vi "Autonomous.vi"() -> ()   [LabVIEW 2025]
doc: "This VI starts when autonomous period begins, and will automatically be terminated when it ends. You can carry out timed or sensor driven operations directly to I/O or to subsystems without needing to return to the caller."
uses:
  <vilib>/Rock Robotics/WPI/ThirdParty/Phoenix-LabVIEW/Pigeon IMU/CTRE_PigeonIMU_TareType.ctl
  <vilib>/Rock Robotics/WPI/Utilities/WPI_GetSetVariantRefNum.vi
  <vilib>/Rock Robotics/Network Tables/NT Read String.vi
  Framework/Robot Global Data.vi
  <vilib>/Rock Robotics/Network Tables/NT Read String Array.vi
  <vilib>/Utility/file.llb/Read Delimited Spreadsheet (string).vi
  <vilib>/Rock Robotics/Network Tables/NT Write Numeric Array.vi
panel:
  in  "Is Blue Alliance?":bool
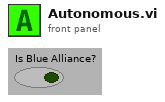
[diagram p1: front panel]
types:
  T1 = typedef "WPI_JoystickDevRef.ctl" = cluster{"Device":T2}
  T2 = typedef "WPI_JoystickDeviceEnum.ctl" = enum16{"USB 0", "USB 1", "USB 2", "USB 3", "USB 4", "USB 5"}
  T3 = cluster{"Field Centric":bool, "Auto Corretion":bool, "Theta Align":bool}
  T4 = typedef "CTRE_PigeonIMU_TareType.ctl" = u8
  T5 = typedef "Robot Velocities.ctl" = cluster{"X Velocity":dbl, "Y Velocity":dbl, "Rotational \nVelocity":dbl}
  T6 = typedef "Single Cmd Info.ctl" = cluster{"Name":string, "CPTM.DataType":variant, "All Control Values Variant":cluster{"Name":string, "Variant Data":variant}[], "icon full":T7, "icon scaled":T7, "Path":path, "Subsystem Color":u32}
  T7 = typedef "imagedata.ctl" = cluster{"image type":i32, "image depth":i32, "image":u8[], "mask":u8[], "colors":u32[], "Rectangle":cluster{"left":i16, "top":i16, "right":i16, "bottom":i16}}
  T8 = cluster{"Name":string, "vi reference":refnum<vi>, i32[], variant[]}
  T9 = cluster{dbl, "Command out":cluster{"Name":string, "vi reference":refnum<vi>, i32[], variant[]}}
  T10 = cluster{dbl, "Command out":cluster{"Name":string, "vi reference":refnum<vi>, i32[], variant[]}}[]
  T11 = cluster{"Velocities":T5[], "Positions":cluster{"x":dbl, "y":dbl, "th":dbl}[], cluster{dbl, "Command out":cluster{"Name":string, "vi reference":refnum<vi>, i32[], variant[]}}[], "Zero Velocity?":bool[], "dt array":dbl[]}
  T12 = typedef "CTRE_PigeonIMU_DeviceRef.ctl" = cluster{"DeviceStatus":errorcluster, "Device Number":u8, "Type":T13, "Device ID":u32, "Handle":u64, "UsageFrame":u32, "Library Path":path}
  T13 = typedef "CTRE_PigeonIMU_ConnectionType.ctl" = u32
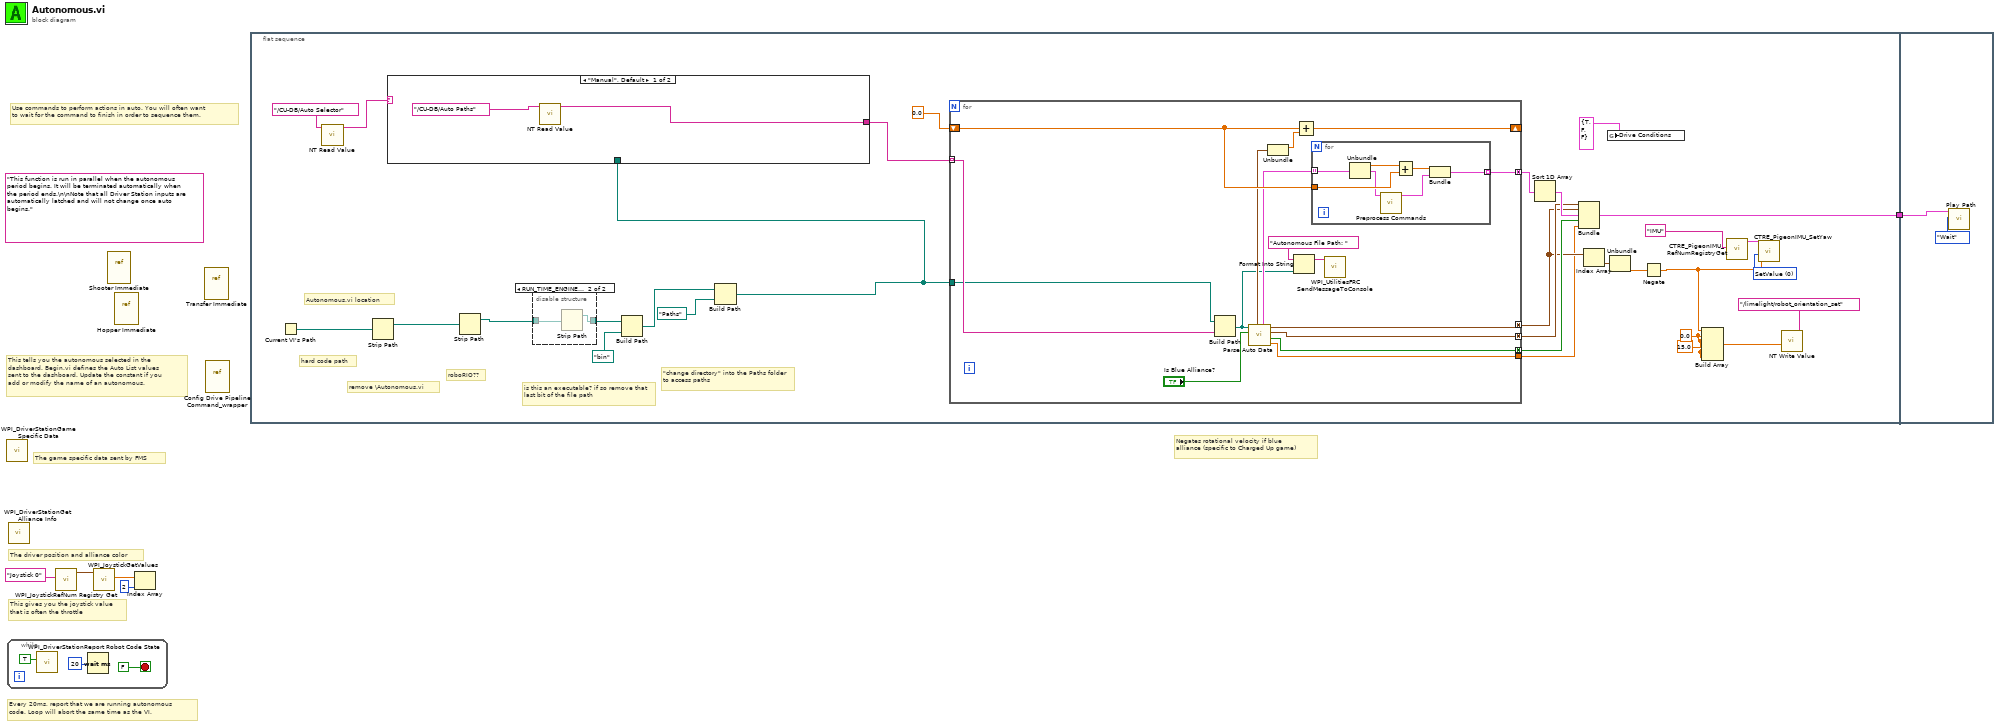
[diagram p0: block diagram]
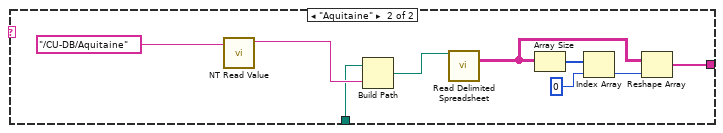
[diagram p3: hidden frame]
diagram:
  (unwired) "This function is run in parallel when the autonomous period begins. It will be terminated automatically when the period ends.\n\nNote that all Driver Station inputs are automatically latched and will not change once auto begins."
  # "Negates rotational velocity if blue alliance (specific to Charged Up game)"
  # "The game specific data sent by FMS"
  # "This tells you the autonomous selected in the \ndashboard. Begin.vi defines the Auto List values\nsent to the dashboard. Update the constant if you\nadd or modify the name of an autonomous."
  # "Every 20ms, report that we are running autonomous\ncode. Loop will abort the same time as the VI."
  # "This gives you the joystick value\nthat is often the throttle"
  # "Use commands to perform actions in auto. You will often want\nto wait for the command to finish in order to sequence them."
  # "The driver position and alliance color"
  n1 = call <vilib>:"WPI_DriverStationGame Specific Data.vi"() -> ()  [unwired: 11 in, 1 out]
  n2 = while {
    stop <- FALSE stop-if-true
    n3 = call <vilib>:"WPI_DriverStationReport Robot Code State.vi"("Autonomous"=TRUE) -> ()  [unwired: 10 in, 1 out]
    n4 = Wait (ms)(milliseconds to wait=u32 20) -> ()  [unwired: 1 out]
  }
  n5 = call <vilib>:"WPI_DriverStationGet Alliance Info.vi"() -> ()  [unwired: 12 out]
  n6 = call <vilib>:"WPI_JoystickRefNum Registry Get.vi"("refnum name"="Joystick 0") -> ("JoystickDevRef"=w4:T1)  [unwired: 1 in, 9 out]
  n7 = call <vilib>:"WPI_JoystickGetValues.vi"("JoystickDevRef"=w4) -> ("Axes"=w3:dbl[])  [unwired: 6 in, 4 out]
  n8 = vi-ref "Shooter Immediate.vi"() -> ()  [unwired: 1 out]
  n9 = vi-ref "Hopper Immediate.vi"() -> ()  [unwired: 1 out]
  n10 = Index Array(array=w3, index=2) -> ()  [unwired: 1 out]
  n11 = vi-ref "Transfer Immediate.vi"() -> ()  [unwired: 1 out]
  n12 = vi-ref "Config Drive Pipeline Command_wrapper.vi"() -> ()  [unwired: 1 out]
  n13 = flat-sequence {
    tunnel: [w19] -> w1
    tunnel: w1 -> [w76]
    frame #0 {
      w12 = T4 0 items=["SetValue"=0, "AddOffset"=1, "MatchCompass"=2, "SetOffset"=255] ("TareType (SetValue)")
      w14 = 0.0 ("element")
      # "\"change directory\" into the Paths folder to access paths"
      # "is this an executable? if so remove that last bit of the file path"
      # "roboRIO??"
      # "remove \\Autonomous.vi"
      # "Autonomous.vi location"
      # "hard code path"
      n14 = Current VI's Path() -> (path=w28:path)
      n15 = call-poly <vilib>:"NT Read Value.vi"("name"="/CU-DB/Auto Selector") -> ("value"=w24:string)  [unwired: 8 in, 2 out]
      n16 = Strip Path(path=w28) -> (stripped path=w29:path)  [unwired: 1 out]
      n17 = Strip Path(path=w29) -> (stripped path=w31:path)  [unwired: 1 out]
      n18 = disable-structure shown="RUN_TIME_ENGINE==True, Default" {
        disable-tunnel: [w39 w40] -> w30
        disable-tunnel: w31 -> [w39 w41]
        frame condition #0 (active) {
        }
        frame condition #1 {
          n19 = Strip Path(path=w41) -> (stripped path=w40:path)  [unwired: 1 out]
        }
      }
      n20 = Build Path(base path=w30, name or relative path=path "bin") -> (appended path=w22:path)
      n21 = Build Path(base path=w22, name or relative path=path "Paths") -> (appended path=w21:path)
      n22 = case shown="\"Manual\", Default" w24 {
        tunnel: w21 -> [_ w73]
        tunnel: [w65 w67] -> w25
        frame "Manual", Default {
          n23 = call-poly <vilib>:"NT Read Value.vi"("name"="/CU-DB/Auto Paths") -> ("value"=w65:string[])  [unwired: 8 in, 2 out]
        }
        frame "Aquitaine" {
          n24 = call-poly <vilib>:"NT Read Value.vi"("name"="/CU-DB/Aquitaine") -> ("value"=w74:string)  [unwired: 8 in, 2 out]
          n25 = Build Path(base path=w73, name or relative path=w74) -> (appended path=w72:path)
          n26 = call-poly <vilib>:"Read Delimited Spreadsheet.vi"("file path (dialog if empty)"=w72) -> ("all rows"=w68:string[][])  [unwired: 9 in, 5 out]
          n27 = Array Size(array=w68) -> (size(s)=w71:i32[])
          n28 = Index Array(array=w71, index=0) -> (element=w69:i32)
          n29 = Reshape Array(w68, w69) -> (w67:string[])
        }
      }
      n30 = for {
        tunnel: [w51] -> w33 mode=concatenating
        tunnel: [w52] -> w32 mode=concatenating
        shift-right: [w57] -> _
        shift-left: 0.0 -> [w55]
        tunnel: [w56] -> w37 mode=concatenating
        tunnel: [w49] -> w34 mode=concatenating
        tunnel: w21 -> [w44]
        tunnel: w25 -> [w45] mode=indexing
        tunnel: [w42] -> w20
        n31 = Build Path(base path=w44, name or relative path=w45) -> (appended path=w48:path)
        n32 = call "Parse Auto Data.vi"("Is Blue Alliance?"="Is Blue Alliance?", "path"=w48) -> ("dt array"=w42:dbl[], "Zero Velocity?"=w49:bool[], "Velocities"=w51:T5[], "Positions"=w52:cluster{"x":dbl, "y":dbl, "th":dbl}[], "Commands out"=w50:cluster{"Time (s)":dbl, T6, bool}[], "Overall"=w54:cluster{"Time (s)":dbl, "Distance (ft)":dbl})  [unwired: 4 in]
        n33 = Unbundle(w54) -> ("Time (s)"=w43:dbl)  [unwired: 1 out]
        n34 = Format Into String(initial string="Autonomous File Path: ", w48) -> (resulting string=w47:string)  [unwired: 2 in, 1 out]
        n35 = Add(x=w55, y=w43) -> (x+y=w57:dbl)
        n36 = for {
          tunnel: w55 -> [w63]
          tunnel: w50 -> [w62] mode=indexing
          tunnel: [w58] -> w56 mode=indexing
          n37 = Unbundle(w62) -> ("Time (s)"=w64:dbl, w61:T6)  [unwired: 1 out]
          n38 = call "Preprocess Commands.vi"("Command In"=w61) -> ("Command out"=w59:T8)  [unwired: 10 in]
          n39 = Add(x=w64, y=w63) -> (x+y=w60:dbl)
          n40 = Bundle(w60, "Command out"=w59) -> (w58:T9)  [unwired: 1 in]
        }
        n41 = call <vilib>:"WPI_UtilitiesFRC SendMessageToConsole.vi"("Message"=w47) -> ()  [unwired: 14 in, 1 out]
      }
      n42 = Sort 1D Array(array=w37) -> (sorted array=w35:T10)
      n43 = Bundle("Velocities"=w33, "Positions"=w32, w35, "Zero Velocity?"=w34, "dt array"=w20) -> (w19:T11)  [unwired: 1 in]
      n44 = Index Array(array=w32) -> (element=w36:cluster{"x":dbl, "y":dbl, "th":dbl})  [unwired: 1 in]
      n45 = global write "Robot Global Data.vi" "Drive Conditions"(T3 {"Field Centric"=TRUE, "Auto Corretion"=FALSE, "Theta Align"=FALSE} ("Drive Conditions")) -> ()
      n46 = Unbundle(w36) -> ("th"=w10:dbl)  [unwired: 2 out]
      n47 = Negate(x=w10) -> (-x=w9:dbl)
      n48 = Build Array(w9, w14, w14, 15.0 ("element"), w14, w14) -> (w13:dbl[])
      n49 = call <vilib>:"CTRE_PigeonIMU_RefNumRegistryGet.vi"("refnum name"="IMU") -> ("PigeonIMUDevRef"=w17:T12)  [unwired: 9 in, 1 out]
      n50 = call <vilib>:"CTRE_PigeonIMU_SetYaw.vi"("TareType (SetValue)"=w12, "Value"=w9, "PigeonIMUDevRef"=w17) -> ()  [unwired: 7 in, 2 out]
      n51 = call-poly <vilib>:"NT Write Value.vi"("value"=w13, "name"="/limelight/robot_orientation_set") -> ()  [unwired: 9 in, 1 out]
    }
    frame #1 {
      n52 = call "Play Path.vi"("Synchronization"=enum16{"Start", "Wait"}."Wait", "Auto Data"=w76) -> ()  [unwired: 9 in, 1 out]
    }
  }
